vi "Open Spark Drive.vi"(5 "Set Master/Slave?":bool, 7 "Set Ramp Rate?":bool, 8 "CAN IDs":u8[](array[numeric]), 10 "Idle Mode":T1, 11 "Full Acceleration Time":sgl) -> ()   [LabVIEW 2018]
uses:
  <vilib>/Rock Robotics/WPI/ThirdParty/REV Robotics/SPARK MAX/Typedef/Spark MAX Idle Mode.ctl
  <vilib>/Rock Robotics/WPI/SafetyOutput/WPI_SafetyOutputConfigMenu.ctl
  <vilib>/Rock Robotics/WPI/RobotDrive/WPI_RobotDriveOpen2MotorWithExistingMotors.vi
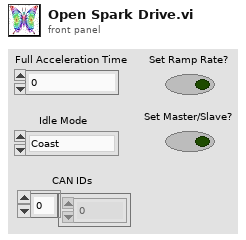
[diagram p1: front panel]
types:
  T1 = typedef "Spark MAX Idle Mode.ctl" = enum16{"Coast", "Brake"}
  T2 = typedef "WPI_MotorControlDeviceRef.ctl" = cluster{"DeviceStatus":errorcluster, "Type":T3, "PWM":cluster{"PWM Channel":T4, "DeadBand":T5}, "CAN":cluster{"Device Number":u8, "SetOutput VI Ref":variant, "GetOutput VI Ref":variant, "Enable VI Ref":variant, "Disable VI Ref":variant, "Data":variant}, "Invert":bool, "DIO PWM":cluster{"PWM \"Enable\" Channel":T4, "DIOChannel":T6, "PWM Rate":dbl}}
  T3 = typedef "WPI_MotorControlType.ctl" = enum16{"PWM", "CAN", "DIO PWM"}
  T4 = typedef "FPGA_DIOPWMChannel.ctl" = enum8{"PWM 0", "PWM 1", "PWM 2", "PWM 3", "PWM 4", "PWM 5", "PWM 6", "PWM 7", "PWM 8", "PWM 9", "PWM MXP 0", "PWM MXP 1", "PWM MXP 2", "PWM MXP 3", "PWM MXP 4", "PWM MXP 5", "PWM MXP 6", "PWM MXP 7", "PWM MXP 8", "PWM MXP 9", "Invalid"}
  T5 = typedef "WPI_PWMDeadband.ctl" = cluster{"Name":string, "maxPositivePwm":i32, "minPositivePwm":i32, "centerPwm":i32, "maxNegativePwm":i32, "minNegativePwm":i32, "angularRange":u16}
  T6 = typedef "FPGA_DIOChannel.ctl" = enum8{"DIO 0", "DIO 1", "DIO 2", "DIO 3", "DIO 4", "DIO 5", "DIO 6", "DIO 7", "DIO 8", "DIO 9", "DIO MXP 0", "DIO MXP 1", "DIO MXP 2", "DIO MXP 3", "DIO MXP 4", "DIO MXP 5", "DIO MXP 6", "DIO MXP 7", "DIO MXP 8", "DIO MXP 9", "DIO MXP 10", "DIO MXP 11", "DIO MXP 12", "DIO MXP 13", "DIO MXP 14", "DIO MXP 15", "SPI Port CS1", "SPI Port CS2", "SPI Port CS3", "SPI Port MISO", "SPI Port MOSI", "Invalid"}
  T7 = typedef "WPI_SafetyOutputConfigMenu.ctl" = enum16{"Enable", "Disable"}
  T8 = typedef "WPI_RobotDriveDevRef.ctl" = cluster{"DevStatus":errorcluster, "Motors[]":T2[], "Square Inputs":bool, "Max Output":dbl}
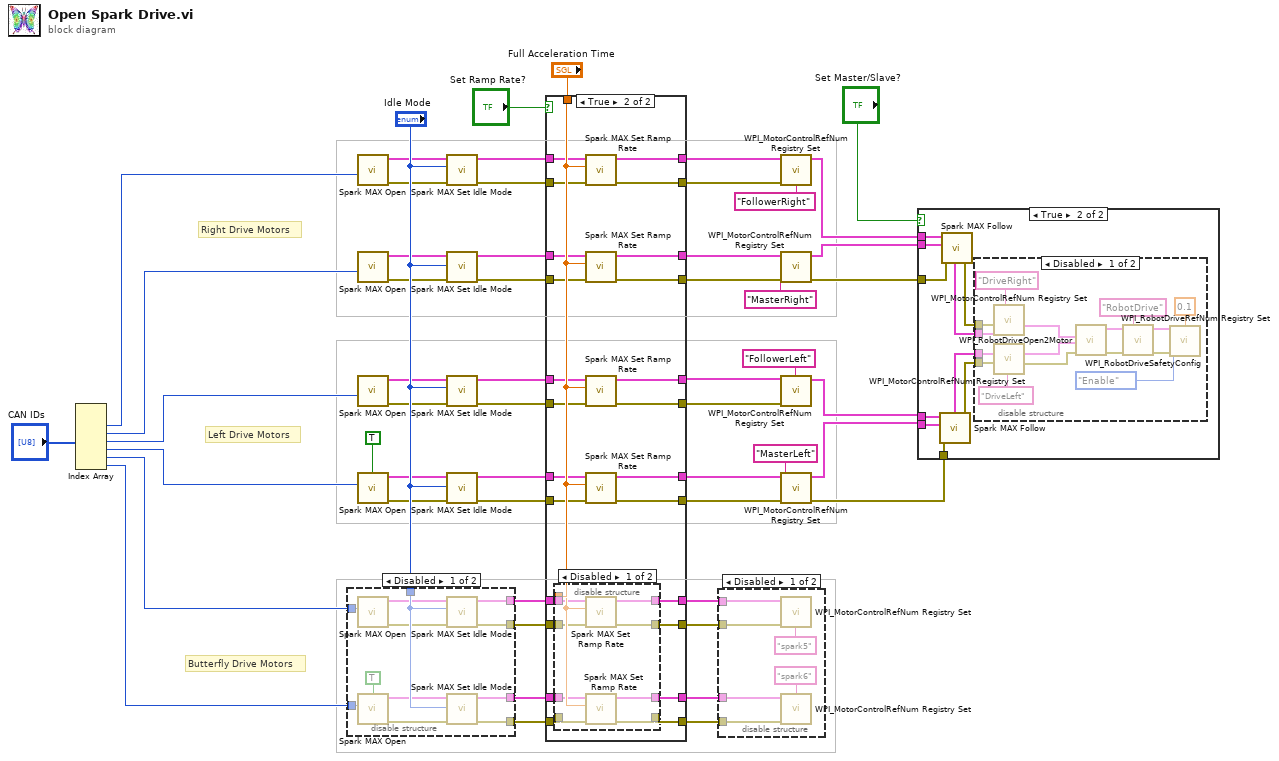
[diagram p0: block diagram]
diagram:
  # "Butterfly Drive Motors"
  # "Left Drive Motors"
  # "Right Drive Motors"
  n1 = Index Array(array="CAN IDs") -> (element #1=w11:u8, element #2=w10:u8, element #3=w9:u8, element #4=w8:u8, element #5=w7:u8, element #6=w6:u8)  [unwired: 6 in]
  n2 = disable-structure shown="Disabled" {
    disable-tunnel: "Idle Mode" -> [w66 _]
    disable-tunnel: [w63 _] -> w46
    disable-tunnel: [w62 _] -> w45
    disable-tunnel: [w60 _] -> w26
    disable-tunnel: [w59 _] -> w24
    disable-tunnel: w7 -> [w57 _]
    disable-tunnel: w6 -> [w56 _]
    frame Disabled {
      n3 = call <vilib>:"Spark MAX Open.vi"("Device Number"=w57) -> ("error out"=w61:errorcluster, "MotorControlDeviceRef"=w65:T2)  [unwired: 9 in]
      n4 = call <vilib>:"Spark MAX Open.vi"("Invert"=TRUE, "Device Number"=w56) -> ("error out"=w58:errorcluster, "MotorControlDeviceRef"=w64:T2)  [unwired: 8 in]
      n5 = call <vilib>:"Spark MAX Set Idle Mode.vi"("error in (no error)"=w61, "Idle Mode"=w66, "MotorControlDeviceRef in"=w65) -> ("error out"=w60:errorcluster, "MotorControlDeviceRef out"=w62:T2)  [unwired: 7 in]
      n6 = call <vilib>:"Spark MAX Set Idle Mode.vi"("error in (no error)"=w58, "Idle Mode"=w66, "MotorControlDeviceRef in"=w64) -> ("error out"=w59:errorcluster, "MotorControlDeviceRef out"=w63:T2)  [unwired: 7 in]
    }
    frame Enabled {
    }
  }
  n7 = call <vilib>:"Spark MAX Open.vi"("Device Number"=w11) -> ("error out"=w35:errorcluster, "MotorControlDeviceRef"=w40:T2)  [unwired: 9 in]
  n8 = call <vilib>:"Spark MAX Open.vi"("Device Number"=w10) -> ("error out"=w33:errorcluster, "MotorControlDeviceRef"=w39:T2)  [unwired: 9 in]
  n9 = call <vilib>:"Spark MAX Open.vi"("Device Number"=w9) -> ("error out"=w31:errorcluster, "MotorControlDeviceRef"=w41:T2)  [unwired: 9 in]
  n10 = call <vilib>:"Spark MAX Open.vi"("Invert"=TRUE, "Device Number"=w8) -> ("error out"=w29:errorcluster, "MotorControlDeviceRef"=w42:T2)  [unwired: 8 in]
  n11 = call <vilib>:"Spark MAX Set Idle Mode.vi"("error in (no error)"=w35, "Idle Mode"="Idle Mode", "MotorControlDeviceRef in"=w40) -> ("error out"=w34:errorcluster, "MotorControlDeviceRef out"=w37:T2)  [unwired: 7 in]
  n12 = call <vilib>:"Spark MAX Set Idle Mode.vi"("error in (no error)"=w33, "Idle Mode"="Idle Mode", "MotorControlDeviceRef in"=w39) -> ("error out"=w32:errorcluster, "MotorControlDeviceRef out"=w38:T2)  [unwired: 7 in]
  n13 = call <vilib>:"Spark MAX Set Idle Mode.vi"("error in (no error)"=w31, "Idle Mode"="Idle Mode", "MotorControlDeviceRef in"=w41) -> ("error out"=w22:errorcluster, "MotorControlDeviceRef out"=w44:T2)  [unwired: 7 in]
  n14 = call <vilib>:"Spark MAX Set Idle Mode.vi"("error in (no error)"=w29, "Idle Mode"="Idle Mode", "MotorControlDeviceRef in"=w42) -> ("error out"=w28:errorcluster, "MotorControlDeviceRef out"=w43:T2)  [unwired: 7 in]
  n15 = case shown="True" "Set Ramp Rate?" {
    tunnel: [w68 w103] -> w54
    tunnel: [w70 w102] -> w53
    tunnel: [w72 w101] -> w52
    tunnel: [w74 w100] -> w51
    tunnel: [w78 w99] -> w50
    tunnel: [w76 w98] -> w49
    tunnel: "Full Acceleration Time" -> [_ w97]
    tunnel: w46 -> [w68 w96]
    tunnel: w45 -> [w70 w95]
    tunnel: w44 -> [w74 w94]
    tunnel: w43 -> [w72 w93]
    tunnel: w38 -> [w76 w92]
    tunnel: w37 -> [w78 w91]
    tunnel: w34 -> [w77 w90]
    tunnel: w32 -> [w75 w89]
    tunnel: [w73 w88] -> w30
    tunnel: w28 -> [w71 w87]
    tunnel: [w71 w86] -> w27
    tunnel: w26 -> [w69 w85]
    tunnel: [w69 w84] -> w25
    tunnel: w24 -> [w67 w83]
    tunnel: [w67 w82] -> w23
    tunnel: w22 -> [w73 w81]
    tunnel: [w75 w80] -> w21
    tunnel: [w77 w79] -> w20
    frame False {
    }
    frame True {
      n16 = disable-structure shown="Disabled" {
        disable-tunnel: [w112 _] -> w103
        disable-tunnel: [w111 _] -> w102
        disable-tunnel: w97 -> [w110 _]
        disable-tunnel: w96 -> [w109 _]
        disable-tunnel: w95 -> [w108 _]
        disable-tunnel: w85 -> [w107 _]
        disable-tunnel: [w106 _] -> w84
        disable-tunnel: w83 -> [w105 _]
        disable-tunnel: [w104 _] -> w82
        frame Disabled {
          n17 = call <vilib>:"Spark MAX Set Ramp Rate.vi"("error in (no error)"=w107, "Seconds from neutral to full (0)"=w110, "MotorControlDeviceRef in"=w108) -> ("error out"=w106:errorcluster, "MotorControlDeviceRef"=w111:T2)  [unwired: 7 in]
          n18 = call <vilib>:"Spark MAX Set Ramp Rate.vi"("error in (no error)"=w105, "Seconds from neutral to full (0)"=w110, "MotorControlDeviceRef in"=w109) -> ("error out"=w104:errorcluster, "MotorControlDeviceRef"=w112:T2)  [unwired: 7 in]
        }
        frame Enabled {
        }
      }
      n19 = call <vilib>:"Spark MAX Set Ramp Rate.vi"("error in (no error)"=w90, "Seconds from neutral to full (0)"=w97, "MotorControlDeviceRef in"=w91) -> ("error out"=w79:errorcluster, "MotorControlDeviceRef"=w99:T2)  [unwired: 7 in]
      n20 = call <vilib>:"Spark MAX Set Ramp Rate.vi"("error in (no error)"=w89, "Seconds from neutral to full (0)"=w97, "MotorControlDeviceRef in"=w92) -> ("error out"=w80:errorcluster, "MotorControlDeviceRef"=w98:T2)  [unwired: 7 in]
      n21 = call <vilib>:"Spark MAX Set Ramp Rate.vi"("error in (no error)"=w81, "Seconds from neutral to full (0)"=w97, "MotorControlDeviceRef in"=w94) -> ("error out"=w88:errorcluster, "MotorControlDeviceRef"=w100:T2)  [unwired: 7 in]
      n22 = call <vilib>:"Spark MAX Set Ramp Rate.vi"("error in (no error)"=w87, "Seconds from neutral to full (0)"=w97, "MotorControlDeviceRef in"=w93) -> ("error out"=w86:errorcluster, "MotorControlDeviceRef"=w101:T2)  [unwired: 7 in]
    }
  }
  n23 = disable-structure shown="Disabled" {
    disable-tunnel: w54 -> [w118 _]
    disable-tunnel: w53 -> [w117 _]
    disable-tunnel: w25 -> [w116 _]
    disable-tunnel: w23 -> [w115 _]
    frame Disabled {
      n24 = call <vilib>:"WPI_MotorControlRefNum Registry Set.vi"("error in (no error)"=w116, "refnum name"="spark5", "MotorControlDevRef"=w117) -> ()  [unwired: 7 in, 2 out]
      n25 = call <vilib>:"WPI_MotorControlRefNum Registry Set.vi"("error in (no error)"=w115, "refnum name"="spark6", "MotorControlDevRef"=w118) -> ()  [unwired: 7 in, 2 out]
    }
    frame Enabled {
    }
  }
  n26 = call <vilib>:"WPI_MotorControlRefNum Registry Set.vi"("error in (no error)"=w20, "refnum name"="FollowerRight" ("string"), "MotorControlDevRef"=w50) -> ("MotorControlDevRef"=w5:T2)  [unwired: 7 in, 1 out]
  n27 = call <vilib>:"WPI_MotorControlRefNum Registry Set.vi"("error in (no error)"=w21, "refnum name"="MasterRight", "MotorControlDevRef"=w49) -> ("error out"=w15:errorcluster, "MotorControlDevRef"=w4:T2)  [unwired: 7 in]
  n28 = call <vilib>:"WPI_MotorControlRefNum Registry Set.vi"("error in (no error)"=w30, "refnum name"="FollowerLeft", "MotorControlDevRef"=w51) -> ("MotorControlDevRef"=w3:T2)  [unwired: 7 in, 1 out]
  n29 = call <vilib>:"WPI_MotorControlRefNum Registry Set.vi"("error in (no error)"=w27, "refnum name"="MasterLeft", "MotorControlDevRef"=w52) -> ("error out"=w16:errorcluster, "MotorControlDevRef"=w2:T2)  [unwired: 7 in]
  n30 = case shown="True" "Set Master/Slave?" {
    tunnel: w2 -> [_ w128]
    tunnel: w3 -> [_ w127]
    tunnel: w5 -> [_ w126]
    tunnel: w4 -> [_ w125]
    tunnel: w16 -> [_ w122]
    tunnel: w15 -> [_ w121]
    frame False {
    }
    frame True {
      n31 = call <vilib>:"Spark MAX Follow.vi"("error in (no error)"=w122, "Master Controller"=w128, "MotorControlDeviceRef"=w127) -> ("error out"=w119:errorcluster, "MotorControlDeviceRef"=w123:T2)  [unwired: 7 in]
      n32 = call <vilib>:"Spark MAX Follow.vi"("error in (no error)"=w121, "Master Controller"=w125, "MotorControlDeviceRef"=w126) -> ("error out"=w120:errorcluster, "MotorControlDeviceRef"=w124:T2)  [unwired: 7 in]
      n33 = disable-structure shown="Disabled" {
        disable-tunnel: w124 -> [w133 _]
        disable-tunnel: w123 -> [w132 _]
        disable-tunnel: w120 -> [w131 _]
        disable-tunnel: w119 -> [w130 _]
        frame Disabled {
          n34 = call <vilib>:"WPI_MotorControlRefNum Registry Set.vi"("error in (no error)"=w131, "refnum name"="DriveRight", "MotorControlDevRef"=w133) -> ("MotorControlDevRef"=w134:T2)  [unwired: 7 in, 1 out]
          n35 = call <vilib>:"WPI_MotorControlRefNum Registry Set.vi"("error in (no error)"=w130, "refnum name"="DriveLeft", "MotorControlDevRef"=w132) -> ("error out"=w129:errorcluster, "MotorControlDevRef"=w135:T2)  [unwired: 7 in]
          n36 = call-poly <vilib>:"WPI_RobotDriveOpen2Motor.vi"("error in (no error)"=w129, "Right Motor Dev Ref"=w134, "Left Motor Dev Ref"=w135) -> ("error out"=w142:errorcluster, "RobotDriveDevRef"=w138:T8)  [unwired: 7 in]
          n37 = call <vilib>:"WPI_RobotDriveRefNum Registry Set.vi"("error in (no error)"=w142, "refnum name"="RobotDrive", "RobotDriveDevRef"=w138) -> ("error out"=w140:errorcluster, "RobotDriveDevRef"=w141:T8)  [unwired: 7 in]
          n38 = call <vilib>:"WPI_RobotDriveSafetyConfig.vi"("error in (no error)"=w140, "timeout (s)"=0.1, "mode"=WPI_SafetyOutputConfigMenu."Enable", "RobotDriveDevRef"=w141) -> ()  [unwired: 6 in, 2 out]
        }
        frame Enabled {
        }
      }
    }
  }
